vi "Transform Object Point by Transformation Matrix.vi"(8 "error in (no error)":errorcluster, 9 "Transformation Matrix (4x4)":T2, 11 "Object Point":T1) -> (0 "error out":errorcluster, 3 "Transformed Point":T1)   [LabVIEW 2020, in "g_ar_toolkit.common.lvlib"]
uses:
  g_ar_toolkit.common/g_ar_toolkit.common.lvlib
  <vilib>/Analysis/Matrix/Datatypes/RealMatrix.ctl
  g_ar_toolkit.common/Object Point (Float).ctl
  <vilib>/Analysis/NI_AALBase.lvlib
  <vilib>/Analysis/Matrix/NI_Matrix.lvlib
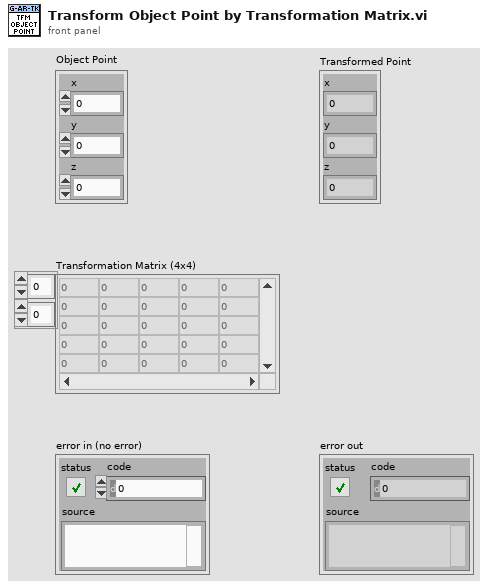
[diagram p1: front panel]
types:
  T1 = typedef "g_ar_toolkit.common.lvlib/Object Point (Float).ctl" = cluster{"x":dbl, "y":dbl, "z":dbl}
  T2 = typedef "NI_Matrix.lvlib/RealMatrix.ctl" = dbl[][]
  T3 = cluster{"A x Vector[0]":dbl, "A x Vector[1]":dbl, "A x Vector[2]":dbl}
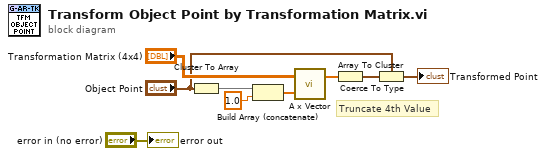
[diagram p0: block diagram]
diagram:
  # "Truncate 4th Value"
  n1 = Cluster To Array(cluster="Object Point") -> (array=w7:dbl[])
  n2 = Build Array (concatenate)(w7, 1.0) -> (w5:dbl[])
  n3 = call <vilib>:"A x Vector.vi"("Vector"=w5, "A"="Transformation Matrix (4x4)") -> ("A x Vector"=w4:dbl[])  [unwired: 1 out]
  n4 = Array To Cluster(array=w4) -> (cluster=w3:T3)
  n5 = Coerce To Type(0:w3, 1:"Object Point") -> (2:→"Transformed Point":T1)
  "error out" <- "error in (no error)"
